vi "Enum info.vi"(8 "error in (no error)":errorcluster, 11 "Variant":variant) -> (0 "error out":errorcluster, 3 "child strings":string[](array[string]))   [LabVIEW 2017, in "DSF Data Viewer.lvlib"]
uses:
  DSF Data Viewer.lvlib
  <vilib>/Utility/Data Type/NI_Data Type.lvlib
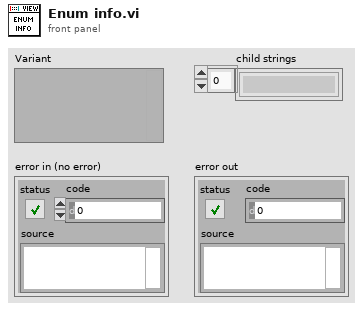
[diagram p1: front panel]
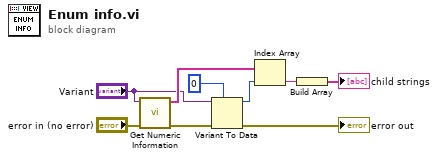
[diagram p0: block diagram]
diagram:
  n1 = call <vilib>:"Get Numeric Information.vi"("error in (no error)"="error in (no error)", "Variant"="Variant") -> ("error out"=w1:errorcluster, "Enum Names"=w5:string[])  [unwired: 6 in, 2 out]
  n2 = Variant To Data(error in=w1, type=u64 0, Variant="Variant") -> (data=w8:u64, error out=→"error out":errorcluster)
  n3 = Index Array(array=w5, index=w8) -> (element=w6:string)
  n4 = Build Array(w6) -> (→"child strings":string[])
